vi "DataFinder_TDMSVIs.vi"() -> ()   [LabVIEW 2023]
doc: "This example executes a query for channel groups in TDMS files. The example uses the VIs \"Create Query\" and \"Executy Query\" to create and execute queries. The example then uses the \"TDMS\" functions to load the mass data of the found channel groups and graphically displays the data."
uses:
  <vilib>/DataFinder/DataTypes/object type.ctl
  <vilib>/DataFinder/DataTypes/comparison operator.ctl
  <vilib>/userdefined/High Color/DFDataFinder.ctl
  <vilib>/DataFinder/Create Query (String).vi
  <vilib>/DataFinder/Close Reference (Results).vi
  <vilib>/DataFinder/Close Reference (Query).vi
  <vilib>/DataFinder/Close Reference (DataFinder).vi
  <vilib>/DataFinder/NI_DataFinder.lvlib
  <vilib>/userdefined/NI_DataFinder Controls.lvlib
panel:
  in  "DataFinder":T1
  in  "Operator":T2 items=["=", "<>", ">", "<", ">=", "<=", "#"]
  in  "Object Type":T3=2 items=["File", "Channel Group", "Channel"]
  in  "Value":string="Temp_A"
  in  "Property Name":string="name"
  out "Results Count":i32 min=0 max=0
  out "Resulting Signals":dynamicdata(graph)
  # "Overview: Uses the DataFinder Toolkit VIs to execute a query in TDMS files and uses the TDMS functions to display the resulting groups.\nRequirements: Select a registered DataFinder which has indexed the TDM Server Demo Data and has optimized the custom properties.\nInstructions:\n1. Ensure that the selected DataFinder is already running.\n2. Specify a Query.\nTo use the predefined search values ensure the folder [all users]\\Documents\\National Instruments\\DataFinder or one of its parent folders is included in your search areas.\n3. Run the VI.\n4. View the Resulting Signals."
  # "Query"
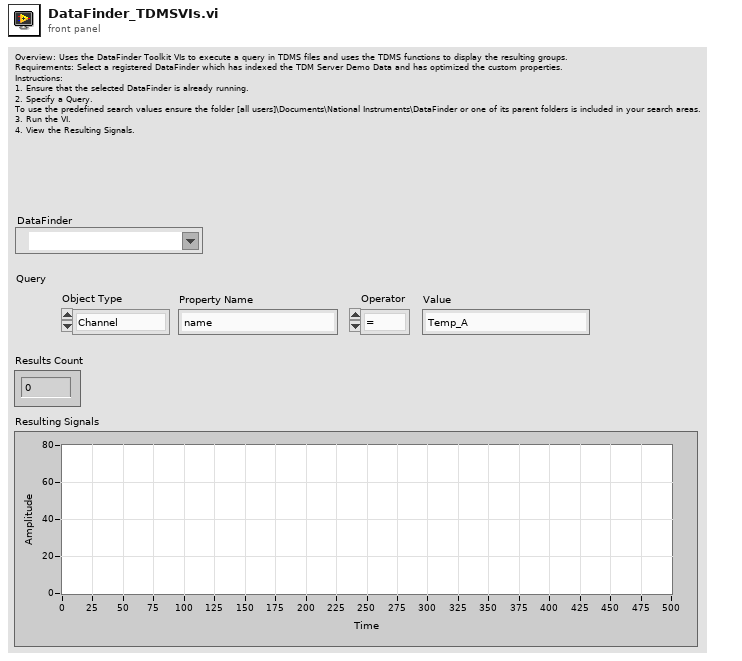
[diagram p1: front panel]
types:
  T1 = typedef "NI_DataFinder Controls.lvlib/DFDataFinder.ctl" = refnum<k21>
  T2 = typedef "NI_DataFinder.lvlib/comparison operator.ctl" = u16
  T3 = typedef "NI_DataFinder.lvlib/object type.ctl" = u16
  T4 = typedef "NI_DataFinder Controls.lvlib/DFQuery.ctl" = refnum<k20>
  T5 = typedef "NI_DataFinder Controls.lvlib/DFSearchResult.ctl" = refnum<k20>
  T6 = typedef "NI_DataFinder.lvlib/results elements.ctl" = cluster{"fullpaths":path[], "DataPlugin names":string[], "channel group names":string[], "channel names":string[]}
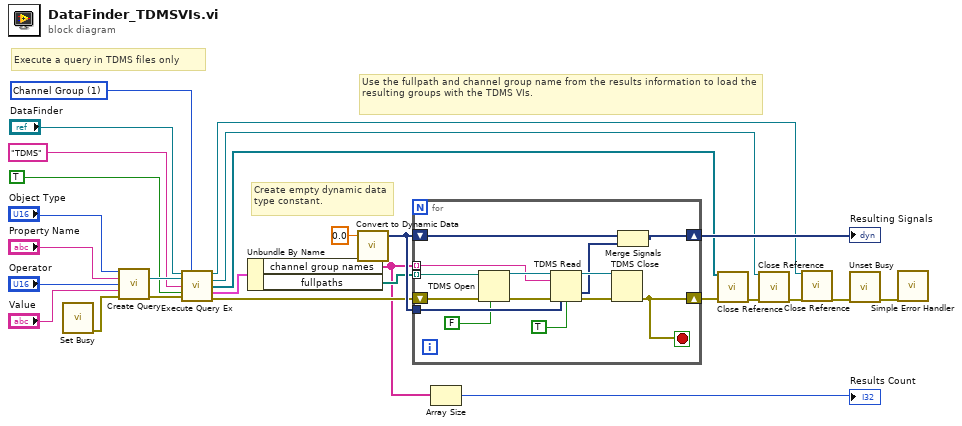
[diagram p0: block diagram]
diagram:
  w18 = T3 1 items=["File", "Channel Group", "Channel"] ("result object type (file)")
  # "Execute a query in TDMS files only"
  # "Create empty dynamic data type constant."
  # "Use the fullpath and channel group name from the results information to load the resulting groups with the TDMS VIs."
  n1 = call <vilib>:"Set Busy.vi"() -> ("error out"=w5:errorcluster)  [unwired: 10 in, 1 out]
  n2 = call-poly <vilib>:"Create Query.vi"("object type"="Object Type", "property name"="Property Name", "comparison operator (=)"="Operator", "value"="Value", "error in (no error)"=w5) -> ("query reference out"=w20:T4, "error out"=w21:errorcluster)  [unwired: 9 in]
  n3 = call <vilib>:"Execute Query Ex.vi"("DataFinder reference"="DataFinder", "result object type (file)"=w18, "query reference"=w20, "DataPlugin name"="TDMS", "fill results elements? (F)"=TRUE, "error in (no error)"=w21) -> ("DataFinder reference out"=w7:T1, "query reference out"=w8:T4, "result references out"=w10:T5[], "results elements"=w15:T6, "error out"=w14:errorcluster)  [unwired: 4 in, 1 out]
  n4 = Unbundle By Name(w15) -> ("channel group names"=w6:string[], "fullpaths"=w13:path[])
  n5 = call "Convert to Dynamic Data"("Double"=0.0) -> ("Dynamic Data Type"=w24:dynamicdata)  [unwired: 3 out]
  n6 = for {
    shift-right: [w35] -> w26
    shift-left: w24 -> [w34]
    shift-right: [w32] -> w11
    shift-left: w14 -> [w40]
    tunnel: w13 -> [w41] mode=indexing
    tunnel: w24 -> [w36]
    tunnel: w6 -> [w29] mode=indexing
    stop <- w32 stop-if-true
    n7 = TDMS Open(6:FALSE ("disable buffering (T)"), 8:w40, 11:w41) -> (0:w38:errorcluster, 3:w39:refnum<k34>)  [unwired: 4 in]
    n8 = TDMS Read(0:w39, 5:w29, 11:w38, 12:w36, 13:TRUE ("return channels in file order? (F)")) -> (4:w37:refnum<k34>, 10:w33:dynamicdata, 15:w30:errorcluster)  [unwired: 3 in, 3 out]
    n9 = TDMS Close(8:w30, 11:w37) -> (0:w32:errorcluster)  [unwired: 1 out]
    n10 = Merge Signals(w34, w33) -> (w35:dynamicdata)
  }
  "Resulting Signals" <- w26
  n11 = Array Size(array=w6) -> (size(s)=→"Results Count":i32)
  n12 = call-poly <vilib>:"Close Reference.vi"("result references"=w10, "error in (no error)"=w11) -> ("error out"=w12:errorcluster)  [unwired: 13 in]
  n13 = call-poly <vilib>:"Close Reference.vi"("query reference"=w8, "error in (no error)"=w12) -> ("error out"=w9:errorcluster)  [unwired: 13 in]
  n14 = call-poly <vilib>:"Close Reference.vi"("DataFinder reference"=w7, "error in (no error)"=w9) -> ("error out"=w4:errorcluster)  [unwired: 13 in]
  n15 = call <vilib>:"Unset Busy.vi"("error in (no error)"=w4) -> ("error out"=w3:errorcluster)  [unwired: 10 in]
  n16 = call <vilib>:"Simple Error Handler.vi"("error in (no error)"=w3) -> ()  [unwired: 4 in, 5 out]
